vi "_wmg_4booltonum.vi"(1 "input4":bool=TRUE, 2 "input3":bool=TRUE, 3 "input2":bool=TRUE, 4 "input1":bool=TRUE) -> (0 "output":i16)   [LabVIEW 2011]
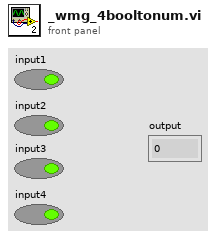
[diagram p1: front panel]
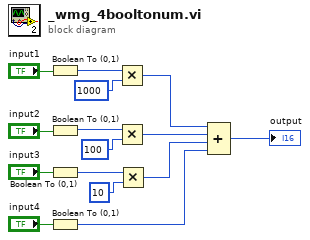
[diagram p0: block diagram]
diagram:
  n1 = Boolean To (0,1)(Boolean="input1") -> (0, 1=w11:i16)
  n2 = Boolean To (0,1)(Boolean="input2") -> (0, 1=w8:i16)
  n3 = Boolean To (0,1)(Boolean="input3") -> (0, 1=w6:i16)
  n4 = Boolean To (0,1)(Boolean="input4") -> (0, 1=w2:i16)
  n5 = Multiply(x=w11, y=i16 1000) -> (x*y=w5:i16)
  n6 = Multiply(x=w8, y=i16 100) -> (x*y=w4:i16)
  n7 = Multiply(x=w6, y=i16 10) -> (x*y=w3:i16)
  n8 = Compound Arithmetic op=ADD(w5, w4, w3, w2) -> (→"output":i16)
